vi "策略模式DEMO.vi"() -> ()   [LabVIEW 2013]
uses:
  Strategy_class/Strategy.lvclass
  <vilib>/addons/_AddQ/G#Object/G#Object.lvclass
  Add_class/Add.lvclass
  Mul_class/Mul.lvclass
panel:
  in  "Operation":enum16{"Add", "Mul"}(ring)
  in  "停止":bool
  out "# of objects killed":i32
  out "Output":string
  out "result":dbl
  in  "y":dbl
  in  "x":dbl
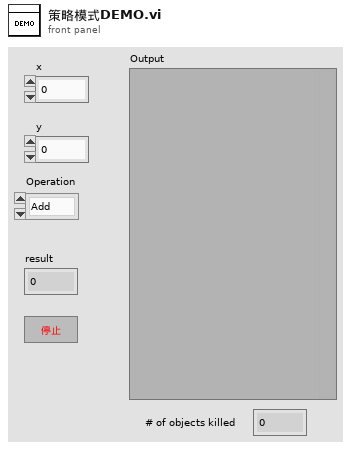
[diagram p1: front panel]
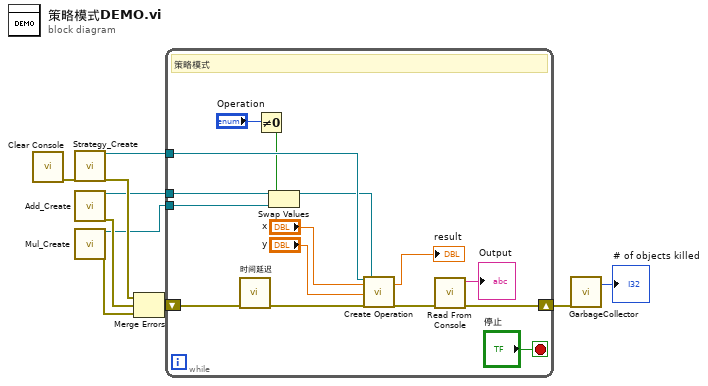
[diagram p0: block diagram]
diagram:
  n1 = call "Clear Console.vi"() -> ("error out"=w8:errorcluster)  [unwired: 11 in]
  n2 = call "Strategy_Create.vi"("error in (no error)"=w8) -> ("reference out"=w3:refnum<class "Strategy.lvclass">, "error out"=w7:errorcluster)  [unwired: 17 in]
  n3 = call "Add_Create.vi"() -> ("reference out"=w2:refnum<class "Add.lvclass">, "error out"=w6:errorcluster)  [unwired: 18 in]
  n4 = call "Mul_Create.vi"() -> ("reference out"=w1:refnum<class "Mul.lvclass">, "error out"=w5:errorcluster)  [unwired: 18 in]
  n5 = Merge Errors(w7, w6, w5) -> (w4:errorcluster)
  n6 = while {
    shift-right: [w24] -> w10
    shift-left: w4 -> [w25]
    tunnel: w3 -> [w16]
    tunnel: w2 -> [w14]
    tunnel: w1 -> [w12]
    stop <- "停止" stop-if-true
    # "策略模式"
    n7 = call "时间延迟"("error in (no error)"=w25) -> ("error out"=w21:errorcluster)  [unwired: 10 in]
    n8 = Not Equal To 0?(x="Operation") -> (x != 0?=w13:bool)
    n9 = Swap Values(12:w14, 13:w13, 14:w12) -> (1:w11:refnum<class "Operation.lvclass">)  [unwired: 1 out]
    n10 = call-dynamic "Create Operation.vi"("reference in"=w16, "x"="x", "y"="y", "error in (no error)"=w21, "Operation.lvclass"=w11) -> ("result"=→"result":dbl, "error out"=w17:errorcluster)  [unwired: 12 in, 1 out]
    n11 = call "Read From Console.vi"("error in (no error)"=w17) -> ("error out"=w24:errorcluster, "Output"=→"Output":string)  [unwired: 9 in]
  }
  n12 = call <vilib>:"GarbageCollector.vi"("error in (no error)"=w10) -> ("# of objects killed"=→"# of objects killed":i32)  [unwired: 16 in, 2 out]
